vi "Guardado.vi"(0 "Tiempo":dbl[](array[numeric]) format="%.2f", 1 "Log_Time":dbl[](array[numeric]) format="%.2f", 2 "Raiz_Time":dbl[](array[numeric]) format="%.2f", 3 "Carga":dbl[](array[numeric]) format="%.2f", 4 "LVDT_AX":dbl[](array[numeric]) format="%.2f", 5 "P.Poro":dbl[](array[numeric]) format="%.2f", 6 "Function":T1(ring), 7 "P.Camara":dbl[](array[numeric]) format="%.2f", 8 "Path":path, 9 "LVDT_Vol":dbl[](array[numeric]) format="%.2f", 10 "Boolean":bool, 11 "Etapa":string, 13 "BSkempton":dbl[](array[numeric]) format="%.2f") -> (17 "ArrayOut":dbl[](array[numeric]) format="%.2f")   [LabVIEW 2015]
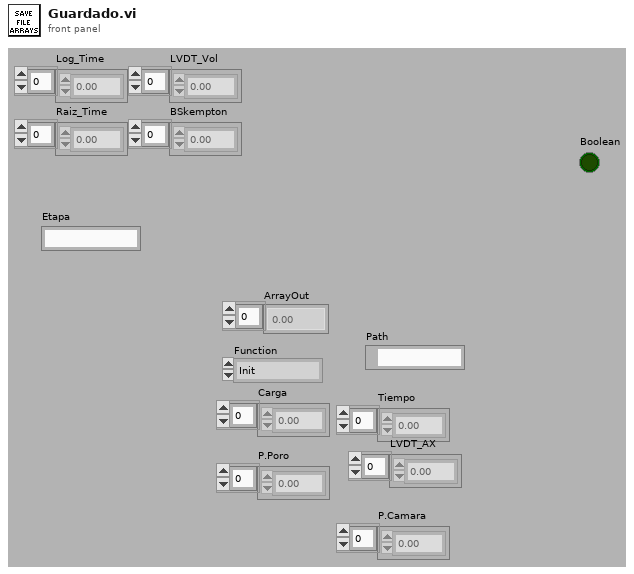
[diagram p1: front panel]
types:
  T1 = enum16{"Init", "Write", "Read array", "Read subarray"}
  T2 = enum16{"open", "open or create", "create or replace", "create", "open (read-only)"}
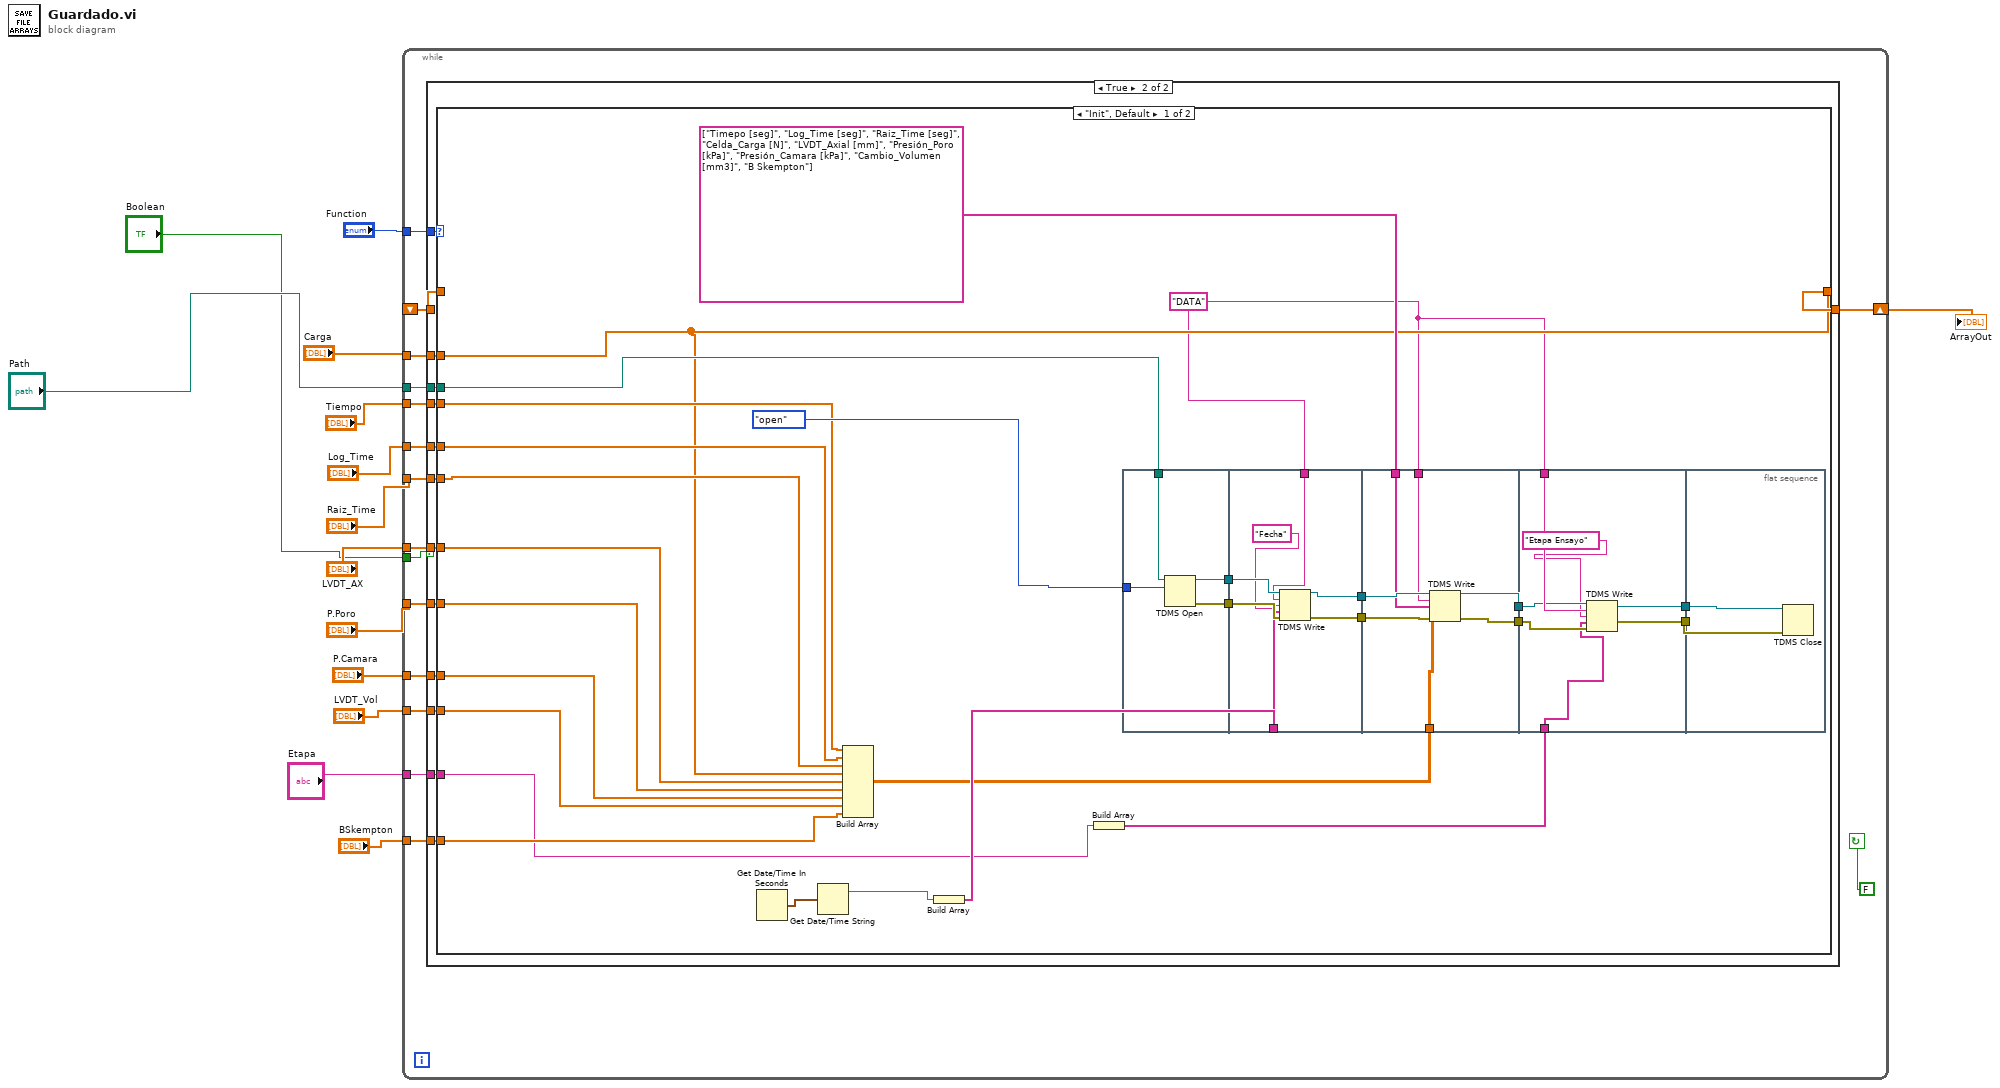
[diagram p0: block diagram]
diagram:
  n1 = while {
    tunnel: "Function" -> [w30]
    shift-right: [w29] -> w12
    shift-left: _ -> [w28]
    tunnel: "Carga" -> [w27]
    tunnel: "Tiempo" -> [w25]
    tunnel: "Log_Time" -> [w24]
    tunnel: "Path" -> [w23]
    tunnel: "Raiz_Time" -> [w22]
    tunnel: "P.Poro" -> [w21]
    tunnel: "LVDT_AX" -> [w20]
    tunnel: "P.Camara" -> [w19]
    tunnel: "LVDT_Vol" -> [w18]
    tunnel: "Etapa" -> [w17]
    tunnel: "BSkempton" -> [w16]
    tunnel: "Boolean" -> [w15]
    stop <- FALSE continue-if-true
    n2 = case shown="True" w15 {
      tunnel: w30 -> [_ w45]
      tunnel: [w31 w44] -> w29
      tunnel: w28 -> [w31 w43]
      tunnel: w27 -> [_ w42]
      tunnel: w25 -> [_ w41]
      tunnel: w24 -> [_ w40]
      tunnel: w23 -> [_ w39]
      tunnel: w22 -> [_ w38]
      tunnel: w21 -> [_ w37]
      tunnel: w20 -> [_ w36]
      tunnel: w19 -> [_ w35]
      tunnel: w18 -> [_ w34]
      tunnel: w17 -> [_ w33]
      tunnel: w16 -> [_ w32]
      frame False {
      }
      frame True {
        n3 = case shown="\"Init\", Default" w45 {
          tunnel: [w58 w100] -> w44
          tunnel: w43 -> [_ w100]
          tunnel: w42 -> [w58 _]
          tunnel: w41 -> [w61 _]
          tunnel: w40 -> [w60 _]
          tunnel: w39 -> [w63 _]
          tunnel: w38 -> [w59 _]
          tunnel: w37 -> [w56 _]
          tunnel: w36 -> [w57 _]
          tunnel: w35 -> [w55 _]
          tunnel: w34 -> [w54 _]
          tunnel: w33 -> [w47 _]
          tunnel: w32 -> [w48 _]
          frame "Init", Default {
            w49 = "DATA"
            n4 = Get Date/Time In Seconds() -> (seconds since 1Jan1904=w68:timestamp)
            n5 = Get Date/Time String(seconds (now)=w68) -> (date string=w64:string)  [unwired: 2 in, 1 out]
            n6 = Build Array(w61, w60, w59, w58, w57, w56, w55, w54, w48) -> (w62:dbl[][])
            n7 = Build Array(w64) -> (w67:string[])
            n8 = Build Array(w47) -> (w46:string[])
            n9 = flat-sequence {
              tunnel: T2."open" ("operation (0:open)") -> [w76]
              tunnel: w63 -> [w75]
              tunnel: [w74] -> w72
              tunnel: [w73] -> w71
              tunnel: w72 -> [w83]
              tunnel: w71 -> [w82]
              tunnel: [w81] -> w70
              tunnel: [w80] -> w69
              tunnel: w49 -> [w78]
              tunnel: w67 -> [w77]
              tunnel: w70 -> [w90]
              tunnel: [w89] -> w53
              tunnel: [w88] -> w51
              tunnel: w69 -> [w87]
              tunnel: w49 -> [w86]
              tunnel: string[] ["Timepo [seg]", "Log_Time [seg]", "Raiz_Time [seg]", "Celda_Carga [N]", "LVDT_Axial [mm]", "Presión_Poro [kPa]", "Presión_Camara [kPa]", "Cambio_Volumen [mm3]", "B Skempton"] ("channel name(s) in (Untitled)") -> [w85]
              tunnel: w62 -> [w84]
              tunnel: w53 -> [w95]
              tunnel: [w94] -> w52
              tunnel: w51 -> [w96]
              tunnel: [w93] -> w50
              tunnel: w49 -> [w97]
              tunnel: w46 -> [w91]
              tunnel: w52 -> [w99]
              tunnel: w50 -> [w98]
              frame #0 {
                n10 = TDMS Open(10:w76, 11:w75) -> (0:w73:errorcluster, 3:w74:refnum<k34>)  [unwired: 5 in]
              }
              frame #1 {
                n11 = TDMS Write(0:w83, 5:w78, 7:"Fecha" ("channel name(s) in (Untitled)"), 9:w77, 11:w82) -> (4:w81:refnum<k34>, 15:w80:errorcluster)  [unwired: 1 in, 2 out]
              }
              frame #2 {
                n12 = TDMS Write(0:w90, 5:w86, 7:w85, 9:w84, 11:w87) -> (4:w89:refnum<k34>, 15:w88:errorcluster)  [unwired: 1 in, 2 out]
              }
              frame #3 {
                n13 = TDMS Write(0:w95, 5:w97, 7:"Etapa Ensayo" ("channel name(s) in (Untitled)"), 9:w91, 11:w96) -> (4:w94:refnum<k34>, 15:w93:errorcluster)  [unwired: 1 in, 2 out]
              }
              frame #4 {
                n14 = TDMS Close(8:w98, 11:w99) -> ()  [unwired: 2 out]
              }
            }
          }
          frame "Read array" {
          }
        }
      }
    }
  }
  "ArrayOut" <- w12
